vi "界面UI.vi"() -> ()   [LabVIEW 2016, in "德润DR803F超标留样.lvlib"]
uses:
  <vilib>/Utility/miscctls.llb/LVPointTypeDef.ctl
  <vilib>/Utility/config.llb/NI_LVConfig.lvlib
panel:
  out "采样瓶数":u16
  out "留样模式":T1(ring)
  out "门状态":enum16{"门关", "门开"}(ring)
  out "仪器时间":timestamp format="%<%Y/%m/%d %H:%M:%S>T"
  out "当前瓶号":u16
  out "采样器状态":enum16{"停止", "运行", "系统初始化"}(ring)
  out "采样器进程":i32(listbox)
  in  "工作进程":u16(ring) items=["清洗管路初始化", "采样瓶位置初始化", "采样瓶排空", "清洗管下降", "采样瓶清洗", "清洗管上升", "外置泵延时", "管路润洗", "进样1", "进样2", "排空管路", "采样瓶位置调整", "待机"]
  out "留样瓶满":bool
  in  "采样瓶排空":bool
  out "超标留样等待时间/s":dbl
  in  "流程停止":bool
  in  "流程启动":bool
  out "流程中":bool
  in  "外控留样设置":bool
  in  "外控留样读取":bool
  in  "设置":bool
  out "VISA resource name":refnum<visa-resource-name>="COM10" caption="VISA资源名称"
  in  "采样模式":enum16{"定时留样", "时间等比", "同步留样", "外控留样", "超标留样"}(ring)
  in  "采样启动":bool
  in  "切换运行":bool
  in  "时间校准":bool
  out "读取缓冲区":string
  out "source":string
  out "通讯":bool
  # "只在待机时启动有效"
  # "德润超标留样803F"
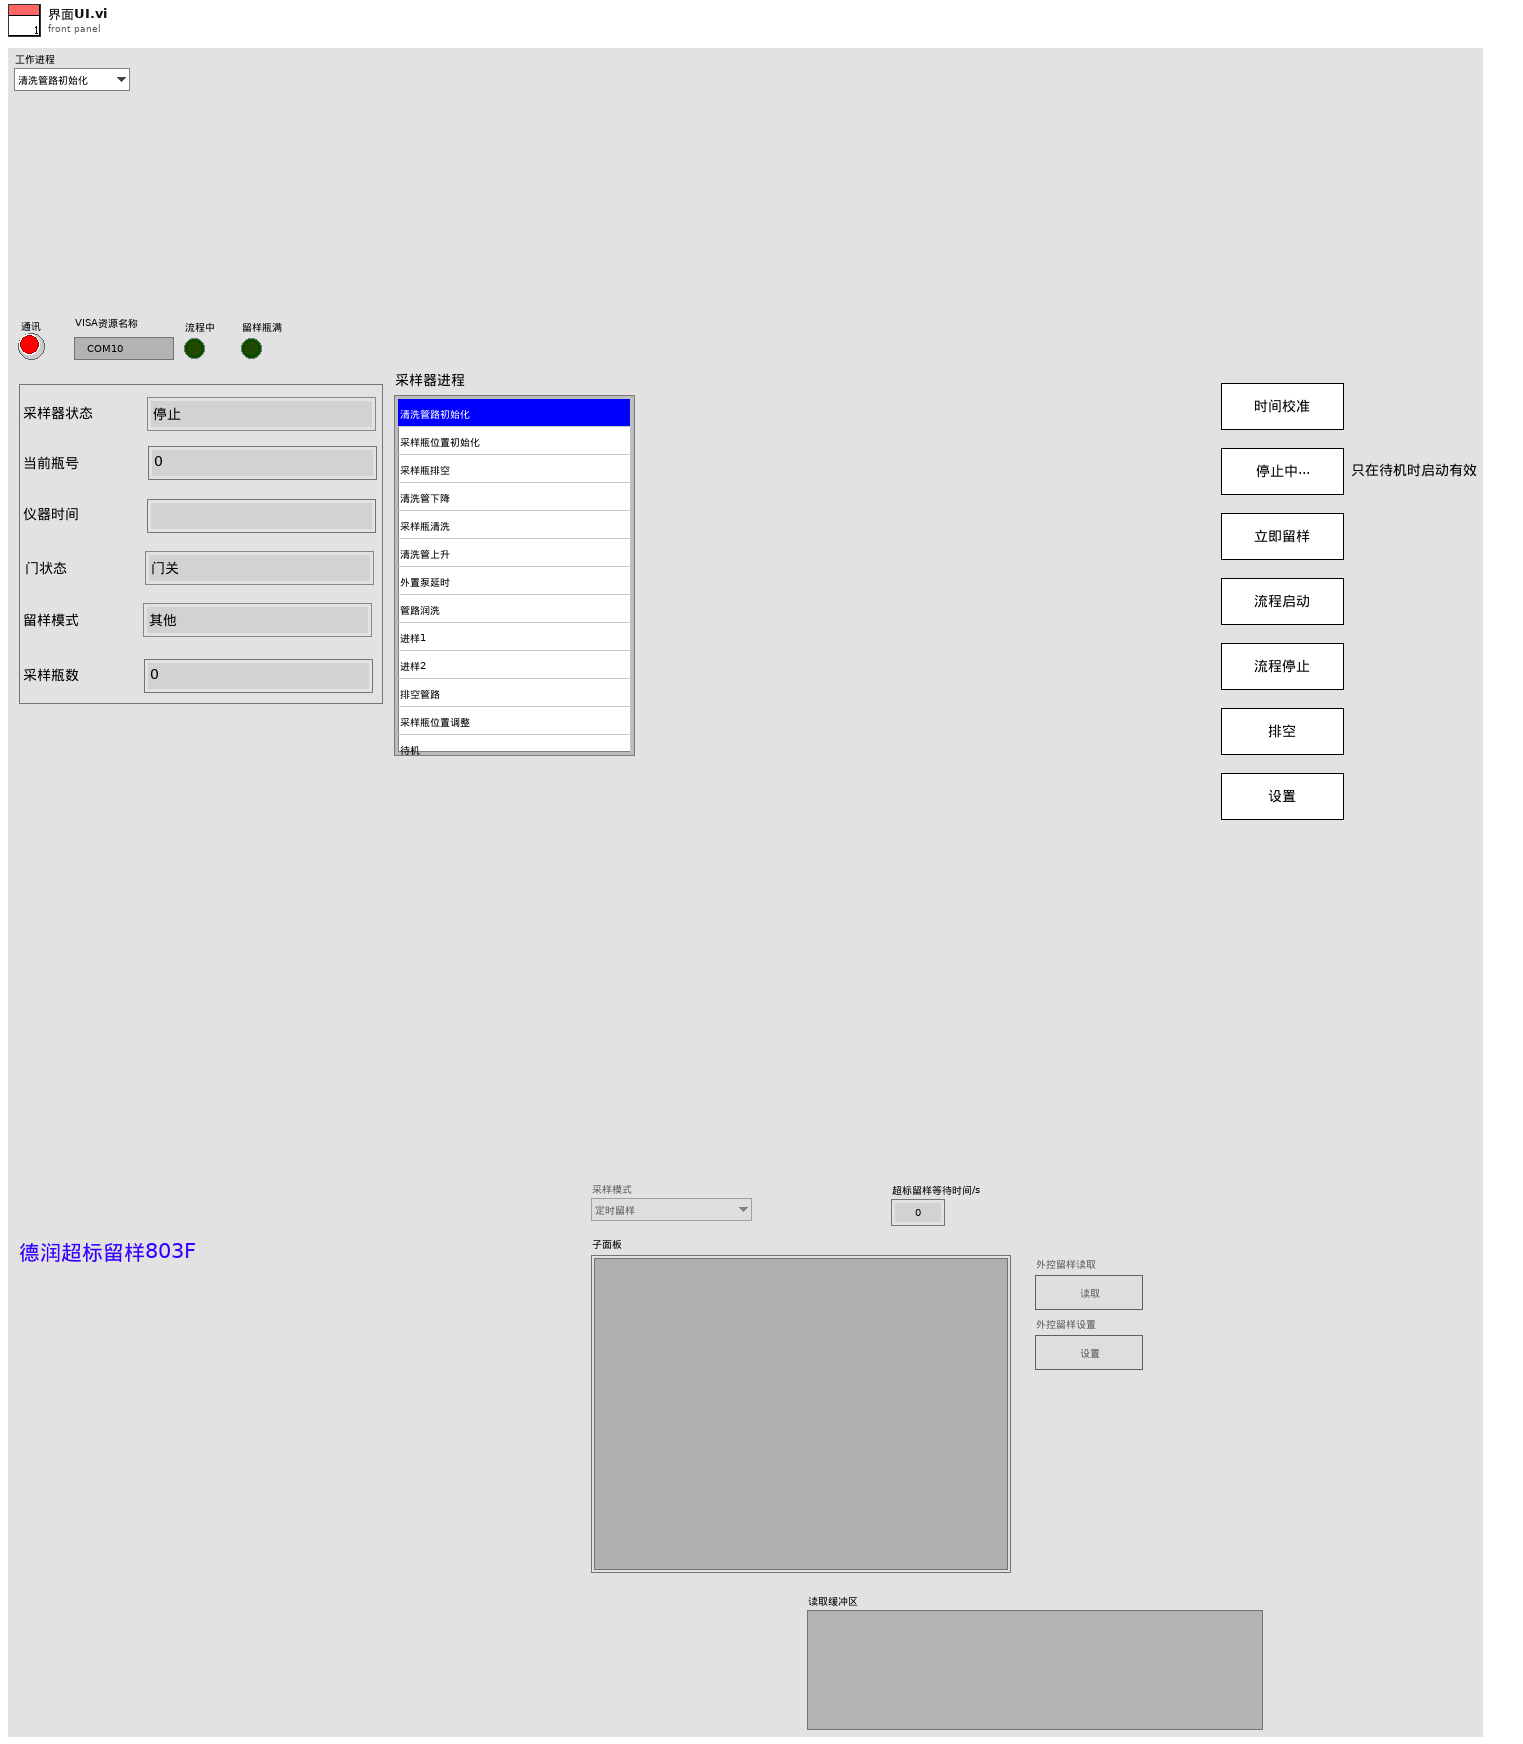
[diagram p1: front panel]
types:
  T1 = enum16{"其他", "定时留样", "时间等比例", "同步留样", "外控留样", "超标留样"}
  T2 = cluster{"枚举":enum16{"open", "read", "write", "close"}, "写入内容":string}
  T3 = cluster{"STEP":enum16{"open", "read", "write", "close"}, "写入缓冲区":string}
  T4 = typedef "LVPointTypeDef.ctl" = cluster{"Horizontal":i16, "Vertical":i16}
  T5 = typedef "NI_LVConfig.lvlib/Config Data RefNum.ctl" = refnum<k1>
  T6 = cluster{"工作状态":u16, "工作进程":u16, "仪器时间":timestamp, "采样模式":u16, "当前瓶号":dbl, "采样瓶数":dbl, "每瓶采样次数":dbl, "当前瓶已采次数":dbl, "当前瓶采样量":dbl, "采样量定量":dbl, "采样量比例":dbl, "瞬时流量":dbl, "累积流量":dbl, "外置泵状态":dbl, "采样泵状态":dbl, "采样泵方向":dbl, "采样阀":dbl, "采样瓶转盘":dbl, "排水阀":dbl, "清洗泵":dbl, "清洗管工作":dbl, "清洗管电源":dbl, "清洗管运行方向":dbl, "门状态":u16, "采水管有水检测":dbl}
  T7 = enum32{"Bad", "Idle", "Run top level", "Running"}
  T8 = cluster{"当前瓶号：":dbl, "平行样：":dbl, "留样瓶数：":dbl, "每瓶次数：":dbl, "每次留样：":dbl}
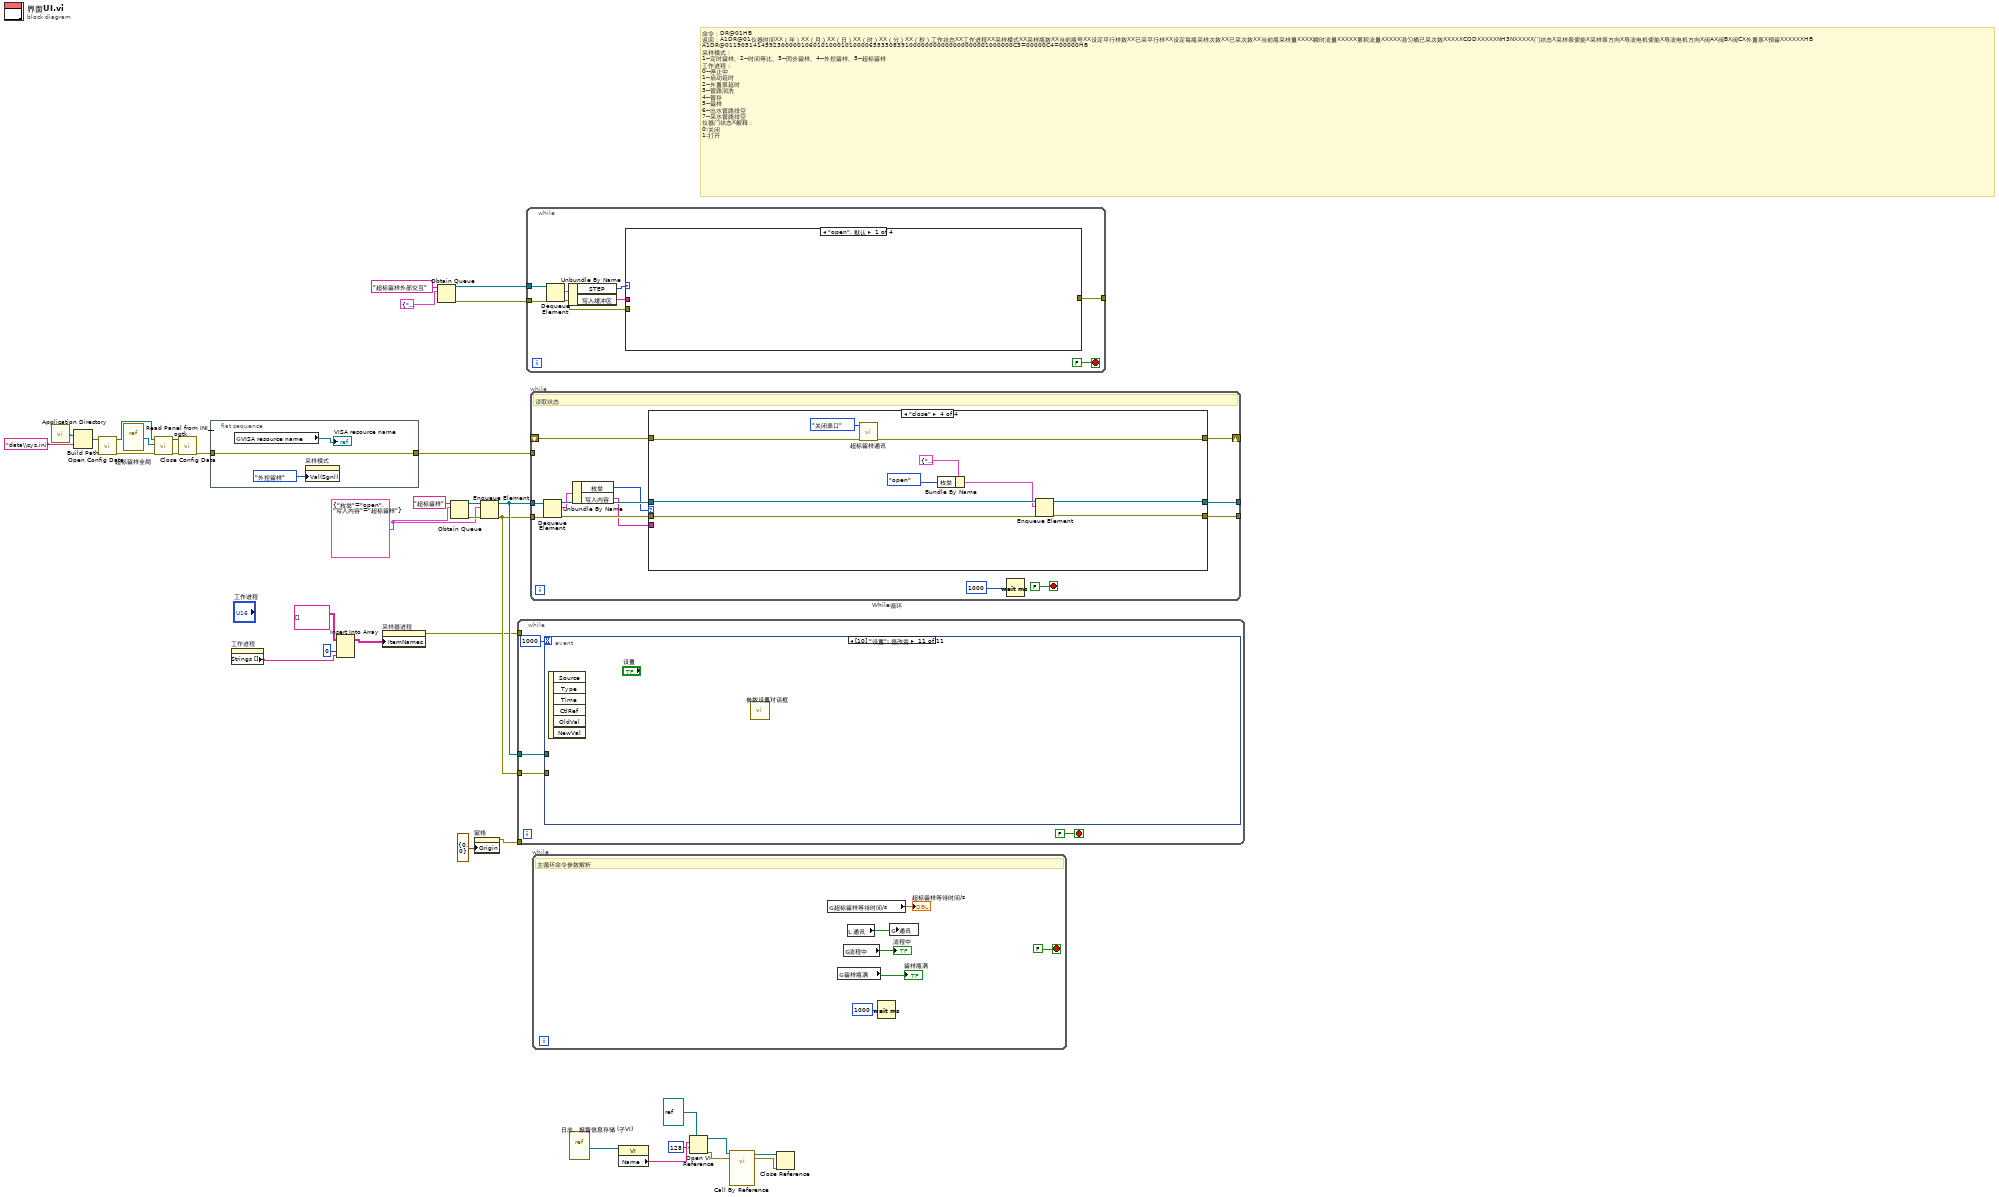
[diagram p0: block diagram]
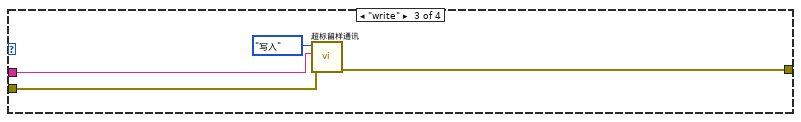
[diagram p3: hidden frame]
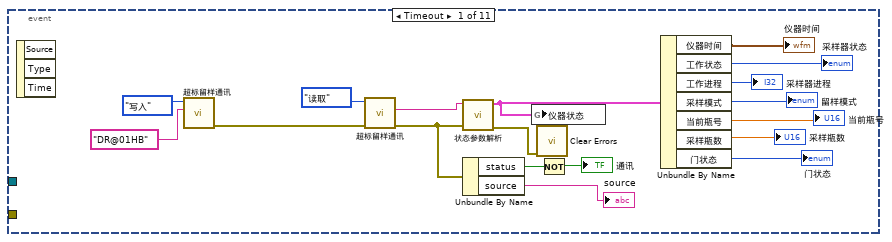
[diagram p5: hidden frame]
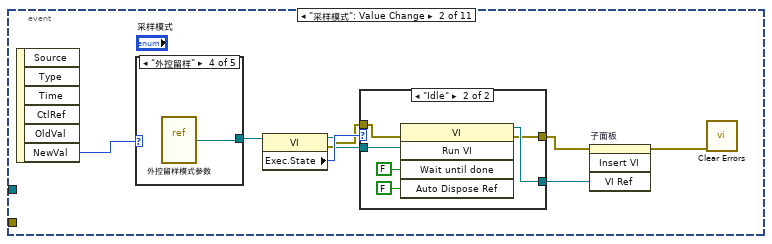
[diagram p6: hidden frame]
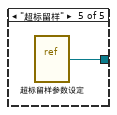
[diagram p11: hidden frame]
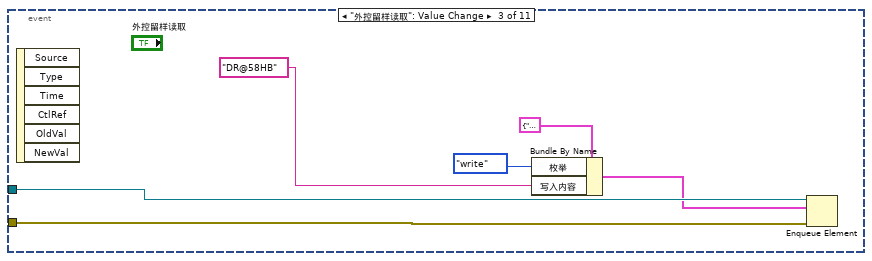
[diagram p12: hidden frame]
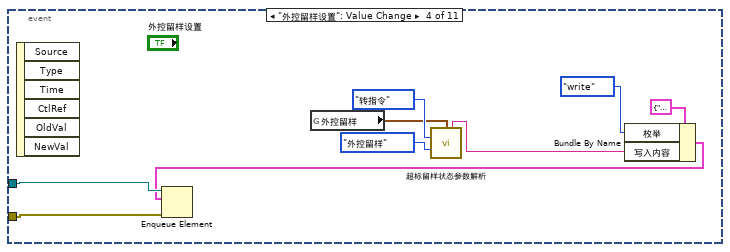
[diagram p13: hidden frame]
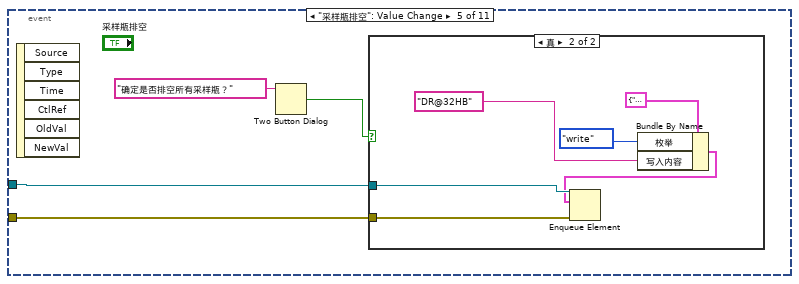
[diagram p14: hidden frame]
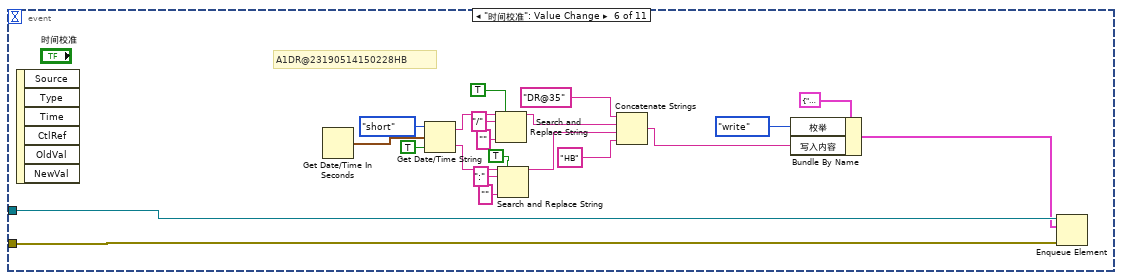
[diagram p16: hidden frame]
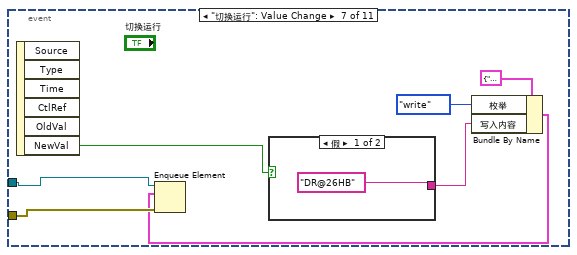
[diagram p17: hidden frame]
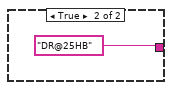
[diagram p18: hidden frame]
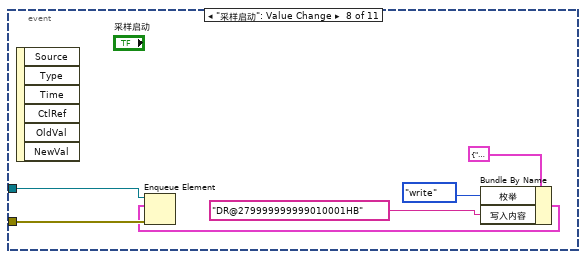
[diagram p19: hidden frame]
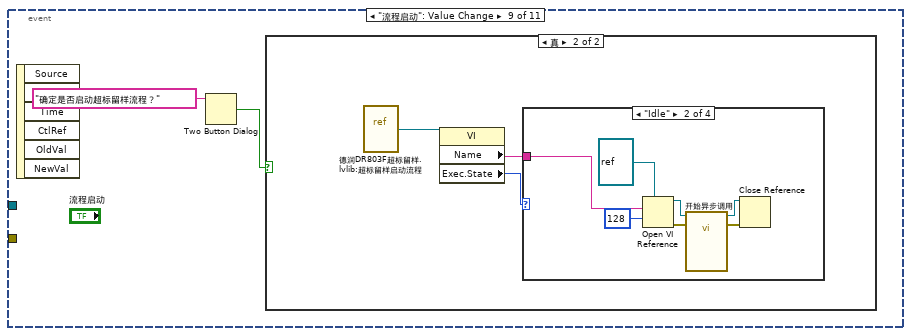
[diagram p20: hidden frame]
diagram:
  w1 = T2 {"枚举"=enum."open", "写入内容"="超标留样"}
  # "命令：DR@01HB\n返回：A1DR@01仪器时间XX（年）XX（月）XX（日）XX（时）XX（分）XX（秒）工作状态XX工作进程XX采样模式XX采样瓶数XX当前瓶号XX设定平行样数XX已采平行样XX设定每瓶采样次数XX已采次数XX当前瓶采样量XXXX瞬时流量XXXXX累积流量XXXXX混匀桶已采次数XXXXXCODXXXXXNH3NXXXXX门状态X采样泵使能X采样泵方向X导流电机使能X导流电机方向X阀AX阀BX阀CX外置泵X预留XXXXXXHB\nA1DR@011905141459230000010601010001010000655350839100000000000000000001000000C3=00000C4=00000HB\n采样模式：\n1--定时留样、2--时间等比、3--同步留样、4--外控留样、5--超标留样\n工作进程：\n0--停止中\n1--启动延时\n2--外置泵延时\n3--管路润洗\n4--管存\n5--留样\n6--出水管路排空\n7--采水管路排空\n仪器门状态X解释：\n0:关闭\n1:打开"
  n1 = call <vilib>:"Application Directory.vi"() -> ("Application Directory"=w29:path)
  n2 = Build Path(base path=w29, name or relative path="data\\sys.ini" ("名称或相对路径")) -> (appended path=w27:path)
  n3 = call <vilib>:"Open Config Data.vi"("configuration file path"=w27) -> ("error out"=w23:errorcluster, "refnum"=w26:T5)  [unwired: 8 in, 1 out]
  n4 = vi-ref "超标留样全局.vi"() -> (w25:refnum<vi>)
  n5 = call <userlib>:"Read Panel from INI__ogtk.vi"("error in (no error)"=w23, "VI ref"=w25, "refnum"=w26) -> ("error out"=w22:errorcluster, "refnum out"=w24:T5)  [unwired: 7 in]
  n6 = call <vilib>:"Close Config Data.vi"("error in (no error)"=w22, "refnum"=w24) -> ("error out"=w21:errorcluster)  [unwired: 8 in, 1 out]
  n7 = flat-sequence {
    tunnel: w21 -> [w38]
    tunnel: [w38] -> w20
    frame #0 {
      n8 = global read "超标留样全局.vi" "VISA resource name"() -> (→"VISA resource name":refnum<visa-resource-name>)
      n9 = property on="采样模式" class="Enum (严格)"("Val(Sgnl)"=enum16{"定时留样", "时间等比", "同步留样", "外控留样", "超标留样"}."外控留样" ("采样模式")) -> ()  [unwired: 2 in, 2 out]
    }
  }
  n10 = property on="工作进程" class="Ring (严格)"() -> ("Strings []"=w4:string[])  [unwired: 2 in, 2 out]
  n11 = Insert Into Array(array=string[][] [] ("字符串[]"), index (col)=0 ("禁用的索引 (列)"), new element=w4) -> (w3:string[][])  [unwired: 1 in]
  n12 = property on="采样器进程" class="MCListbox (严格)"("ItemNames"=w3) -> (error out=w2:errorcluster)  [unwired: 2 in, 1 out]
  n13 = Obtain Queue(name (unnamed)="超标留样外部交互" ("名称（未命名）"), element data type=T3 {"STEP"=enum."write", "写入缓冲区"="ª\u0006\u0000\u0000P`\u00000»"}) -> (queue out=w18:refnum<queue>, error out=w17:errorcluster)  [unwired: 3 in, 1 out]
  n14 = Obtain Queue(name (unnamed)="超标留样" ("名称（未命名）"), element data type=w1) -> (queue out=w34:refnum<queue>, error out=w33:errorcluster)  [unwired: 3 in, 1 out]
  n15 = property on="窗格" class="Pane"("Origin"=T4 {"Horizontal"=0, "Vertical"=0} ("原点")) -> (error out=w7:errorcluster)  [unwired: 2 in, 1 out]
  n16 = Enqueue Element(queue=w34, element=w1, error in (no error)=w33) -> (queue out=w32:refnum<queue>, error out=w31:errorcluster)  [unwired: 1 in, 1 out]
  n17 = while {
    tunnel: w32 -> [w41]
    tunnel: w31 -> [w40]
    tunnel: w7 -> [_]
    tunnel: w2 -> [_]
    stop <- FALSE stop-if-true
    n18 = event shown="[10] \"设置\": 值改变" {
      selector: _ -> [_ _ _ _ _ _ _ _ _ _ _]
      dyn-events: _ -> [_ _ _ _ _ _ _ _ _ _ _]
      timeout: 1000 -> [_ _ _ _ _ _ _ _ _ _ _]
      tunnel: w41 -> [_ _ w83 w93 w97 w124 w131 w139 _ w153 _]
      tunnel: w40 -> [_ _ w84 w92 w96 w123 w130 w138 _ w152 _]
      event Timeout {
        n19 = event-data() -> ()  [unwired: 1 in, 3 out]
        n20 = call "超标留样通讯.vi"("写入缓冲区"="DR@01HB", "功能输入"=enum16{"打开串口", "写入", "读取", "关闭串口"}."写入") -> ("error out"=w60:errorcluster)  [unwired: 7 in, 2 out]
        n21 = call "超标留样通讯.vi"("error in (no error)"=w60, "功能输入"=enum16{"打开串口", "写入", "读取", "关闭串口"}."读取") -> ("error out"=w59:errorcluster, "读取缓冲区"=w58:string)  [unwired: 7 in, 1 out]
        n22 = call "状态参数解析.vi"("error in (no error)"=w59, "字符串"=w58) -> ("error out"=w43:errorcluster, "簇"=w51:T6)  [unwired: 8 in]
        n23 = Unbundle By Name(w59) -> ("status"=w52:bool, "source"=→"source":string)
        n24 = global write "超标留样全局.vi" "仪器状态"(w51) -> ()
        n25 = call <vilib>:"Clear Errors.vi"("error in (no error)"=w43) -> ()  [unwired: 5 in, 2 out]
        n26 = Not(x=w52) -> (.not. x?=→"通讯":bool)
        n27 = Unbundle By Name(w51) -> ("仪器时间"=→"仪器时间":timestamp, "工作状态"=→"采样器状态":u16, "工作进程"=→"采样器进程":u16, "采样模式"=→"留样模式":u16, "当前瓶号"=→"当前瓶号":dbl, "采样瓶数"=→"采样瓶数":dbl, "门状态"=→"门状态":u16)
      }
      event "采样模式": Value Change {
        n28 = event-data() -> ("NewVal"=w68:enum16{"定时留样", "时间等比", "同步留样", "外控留样", "超标留样"})  [unwired: 1 in, 5 out]
        n29 = case shown="\"外控留样\"" w68 {
          tunnel: [_ _ _ w77 w78] -> w67
          frame "定时留样", Default {
          }
          frame "时间等比" {
          }
          frame "同步留样" {
          }
          frame "外控留样" {
            n30 = vi-ref "外控留样模式参数.vi"() -> (w77:refnum<vi>)
          }
          frame "超标留样" {
            n31 = vi-ref "超标留样参数设定.vi"() -> (w78:refnum<vi>)
          }
        }
        n32 = property class="VI"(reference=w67) -> (reference out=w65:refnum<vi>, error out=w63:errorcluster, "Exec.State"=w66:T7)  [unwired: 1 in]
        n33 = case shown="\"Idle\"" w66 {
          tunnel: w65 -> [w70 w76]
          tunnel: [w70 w73] -> w64
          tunnel: w63 -> [w69 w72]
          tunnel: [w69 w71] -> w62
          frame "Bad", Default {
          }
          frame "Idle" {
            n34 = invoke class="VI" method="Run VI"(reference=w76, error in=w72, "Wait until done"=FALSE ("结束前等待"), "Auto Dispose Ref"=FALSE ("自动销毁引用")) -> (reference out=w73:refnum<vi>, error out=w71:errorcluster)  [unwired: 1 in, 3 out]
          }
        }
        n35 = invoke on="子面板" class="SubPnl" method="Insert VI"(error in=w62, "VI Ref"=w64) -> (error out=w61:errorcluster)  [unwired: 2 in, 3 out]
        n36 = call <vilib>:"Clear Errors.vi"("error in (no error)"=w61) -> ()  [unwired: 5 in, 2 out]
      }
      event "外控留样读取": Value Change {
        n37 = event-data() -> ()  [unwired: 1 in, 6 out]
        n38 = Bundle By Name(cluster=T2 {"枚举"=enum."open", "写入内容"="超标留样"}, "枚举"=enum16{"open", "read", "write", "close"}."write" ("元素"), "写入内容"="DR@58HB") -> (w79:T2)
        n39 = Enqueue Element(queue=w83, element=w79, error in (no error)=w84) -> ()  [unwired: 1 in, 3 out]
      }
      event "外控留样设置": Value Change {
        n40 = event-data() -> ()  [unwired: 1 in, 6 out]
        n41 = global read "超标留样全局.vi" "外控留样"() -> (w89:T8)
        n42 = call "超标留样状态参数解析.vi"("外控留样"=w89, "解析/转指令"=enum16{"解析", "转指令"}."转指令", "模式选择"=enum16{"外控留样", "超标留样"}."外控留样") -> ("输出字符串"=w86:string)  [unwired: 11 in, 1 out]
        n43 = Bundle By Name(cluster=T2 {"枚举"=enum."open", "写入内容"="超标留样"}, "枚举"=enum16{"open", "read", "write", "close"}."write" ("元素"), "写入内容"=w86) -> (w85:T2)
        n44 = Enqueue Element(queue=w93, element=w85, error in (no error)=w92) -> ()  [unwired: 1 in, 3 out]
      }
      event "采样瓶排空": Value Change {
        n45 = event-data() -> ()  [unwired: 1 in, 6 out]
        n46 = Two Button Dialog(message="确定是否排空所有采样瓶？" ("消息")) -> (T button?=w94:bool)  [unwired: 2 in]
        n47 = case shown="真" w94 {
          tunnel: w97 -> [_ w103]
          tunnel: w96 -> [_ w102]
          frame False {
          }
          frame True {
            n48 = Bundle By Name(cluster=T2 {"枚举"=enum."open", "写入内容"="超标留样"}, "枚举"=enum16{"open", "read", "write", "close"}."write" ("元素"), "写入内容"="DR@32HB") -> (w98:T2)
            n49 = Enqueue Element(queue=w103, element=w98, error in (no error)=w102) -> ()  [unwired: 1 in, 3 out]
          }
        }
      }
      event "时间校准": Value Change {
        # "A1DR@23190514150228HB"
        n50 = event-data() -> ()  [unwired: 1 in, 6 out]
        n51 = Get Date/Time In Seconds() -> (seconds since 1Jan1904=w119:timestamp)
        n52 = Get Date/Time String(date format (0)=enum16{"short", "long", "abbreviated"}."short" ("日期格式(0)"), seconds (now)=w119, want seconds? (F)=TRUE ("需要秒？(F)")) -> (date string=w118:string, time string=w111:string)
        n53 = Search and Replace String(replace all?=TRUE ("替换全部？(F)"), input string=w118, search string="/" ("搜索字符串"), replace string="" ("替换字符串(\"\")")) -> (result string=w110:string)  [unwired: 4 in, 3 out]
        n54 = Search and Replace String(replace all?=TRUE ("替换全部？(F)"), input string=w111, search string=":" ("搜索字符串"), replace string="" ("替换字符串(\"\")")) -> (result string=w109:string)  [unwired: 4 in, 3 out]
        n55 = Concatenate Strings("DR@35" ("写入缓冲区"), w110, w109, "HB" ("写入缓冲区")) -> (w105:string)
        n56 = Bundle By Name(cluster=T2 {"枚举"=enum."open", "写入内容"="超标留样"}, "枚举"=enum16{"open", "read", "write", "close"}."write" ("元素"), "写入内容"=w105) -> (w104:T2)
        n57 = Enqueue Element(queue=w124, element=w104, error in (no error)=w123) -> ()  [unwired: 1 in, 3 out]
      }
      event "切换运行": Value Change {
        n58 = event-data() -> ("NewVal"=w127:bool)  [unwired: 1 in, 5 out]
        n59 = case shown="假" w127 {
          tunnel: ["DR@26HB" ("写入缓冲区") "DR@25HB"] -> w126
          frame False {
          }
          frame True {
          }
        }
        n60 = Bundle By Name(cluster=T2 {"枚举"=enum."open", "写入内容"="超标留样"}, "枚举"=enum16{"open", "read", "write", "close"}."write" ("元素"), "写入内容"=w126) -> (w125:T2)
        n61 = Enqueue Element(queue=w131, element=w125, error in (no error)=w130) -> ()  [unwired: 1 in, 3 out]
      }
      event "采样启动": Value Change {
        n62 = event-data() -> ()  [unwired: 1 in, 6 out]
        n63 = Bundle By Name(cluster=T2 {"枚举"=enum."open", "写入内容"="超标留样"}, "枚举"=enum16{"open", "read", "write", "close"}."write" ("元素"), "写入内容"="DR@279999999999010001HB") -> (w134:T2)
        n64 = Enqueue Element(queue=w139, element=w134, error in (no error)=w138) -> ()  [unwired: 1 in, 3 out]
      }
      event "流程启动": Value Change {
        n65 = event-data() -> ()  [unwired: 1 in, 6 out]
        n66 = Two Button Dialog(message="确定是否启动超标留样流程？" ("消息")) -> (T button?=w140:bool)  [unwired: 2 in]
        n67 = case shown="真" w140 {
          frame False {
          }
          frame True {
            n68 = vi-ref "德润DR803F超标留样.lvlib:超标留样启动流程.vi"() -> (w142:refnum<vi>)
            n69 = property class="VI"(reference=w142) -> ("Name"=w143:string, "Exec.State"=w144:T7)  [unwired: 1 in, 2 out]
            n70 = case shown="\"Idle\"" w144 {
              tunnel: w143 -> [_ w147 _ _]
              frame "Bad", Default {
              }
              frame "Idle" {
                n71 = Open VI Reference(type specifier VI Refnum (for type only)=refnum<vi> refnum ("类型说明符VI引用句柄（仅用于类型）"), vi path=w147, options=128 ("选项")) -> (vi reference=w151:refnum<vi>, error out=w146:errorcluster)  [unwired: 3 in]
                n72 = call-by-ref "开始异步调用"(reference=w151, error in=w146) -> (reference out=w150:refnum<vi>, error out=w145:errorcluster)  [unwired: 12 in]
                n73 = Close Reference(reference=w150, error in (no error)=w145) -> ()  [unwired: 1 out]
              }
              frame "Run top level" {
              }
              frame "Running" {
              }
            }
          }
        }
      }
      event "流程停止": Value Change {
        n74 = event-data() -> ()  [unwired: 1 in, 6 out]
        n75 = Two Button Dialog(message="确定是否停止超标留样流程并排空当前瓶？" ("消息")) -> (T button?=w154:bool)  [unwired: 2 in]
        n76 = case shown="真" w154 {
          tunnel: w153 -> [_ w161]
          tunnel: w152 -> [_ w160]
          frame False {
          }
          frame True {
            n77 = Obtain Notifier(name (unnamed)="超标留样流程" ("名称（未命名）"), notification data type=FALSE ("采样完成")) -> (notifier out=w166:refnum<notifier>, error out=w165:errorcluster)  [unwired: 2 in, 1 out]
            n78 = Send Notification(notification=TRUE ("通知"), notifier=w166, error in (no error)=w165) -> (notifier out=w163:refnum<notifier>, error out=w162:errorcluster)
            n79 = Release Notifier(notifier=w163, error in (no error)=w162) -> ()  [unwired: 1 in, 3 out]
            n80 = Bundle By Name(cluster=T2 {"枚举"=enum."open", "写入内容"="超标留样"}, "枚举"=enum16{"open", "read", "write", "close"}."write" ("元素"), "写入内容"="DR@26HB" ("写入缓冲区")) -> (w156:T2)
            n81 = Enqueue Element(queue=w161, element=w156, error in (no error)=w160) -> ()  [unwired: 1 in, 3 out]
          }
        }
      }
      event "设置": Value Change {
        n82 = event-data() -> ()  [unwired: 1 in, 6 out]
        n83 = call "参数设置对话框.vi"() -> ()  [unwired: 12 in]
      }
    }
  }
  n84 = while {
    tunnel: w18 -> [w176]
    tunnel: w17 -> [w175]
    tunnel: [w169] -> _
    stop <- FALSE stop-if-true
    n85 = Dequeue Element(queue=w176, error in (no error)=w175) -> (element=w173:T3, error out=w170:errorcluster)  [unwired: 1 in, 2 out]
    n86 = Unbundle By Name(w173) -> ("STEP"=w172:enum16{"open", "read", "write", "close"}, "写入缓冲区"=w171:string)
    n87 = case shown="\"open\", 默认" w172 {
      tunnel: w171 -> [_ _ w180 _]
      tunnel: w170 -> [_ _ w178 _]
      tunnel: [_ _ w177 _] -> w169
      frame "open", Default {
      }
      frame "read" {
      }
      frame "write" {
        n88 = call "超标留样通讯.vi"("error in (no error)"=w178, "写入缓冲区"=w180, "功能输入"=enum16{"打开串口", "写入", "读取", "关闭串口"}."写入") -> ("error out"=w177:errorcluster)  [unwired: 6 in, 2 out]
      }
      frame "close" {
      }
    }
  }
  n89 = while "While循环" {
    tunnel: w32 -> [w191]
    tunnel: w31 -> [w190]
    tunnel: [w187] -> _
    tunnel: [w186] -> _
    shift-right: [w184] -> _
    shift-left: _ -> [w185]
    tunnel: w20 -> [_]
    stop <- FALSE stop-if-true
    # "读取状态"
    n90 = Dequeue Element(queue=w191, error in (no error)=w190) -> (queue out=w189:refnum<queue>, element=w183:T2, error out=w188:errorcluster)  [unwired: 1 in, 1 out]
    n91 = Unbundle By Name(w183) -> ("枚举"=w182:enum16{"open", "read", "write", "close"}, "写入内容"=w181:string)
    n92 = case shown="\"close\"" w182 {
      tunnel: [w197 w200 w225 w238] -> w184
      tunnel: w189 -> [w196 w203 w230 w237]
      tunnel: w188 -> [w195 w202 w229 w236]
      tunnel: [w196 w203 w228 w235] -> w187
      tunnel: [w195 w202 w227 w234] -> w186
      tunnel: w185 -> [_ w205 w226 w240]
      tunnel: w181 -> [_ w199 w221 _]
      frame "open", Default {
        (unwired) refnum<visa-resource-name> "COM2" ("VISA resource name")
        n93 = global read "超标留样全局.vi" "VISA resource name"() -> (w194:refnum<visa-resource-name>)
        n94 = call "超标留样通讯.vi"("VISA resource name"=w194, "功能输入"=enum16{"打开串口", "写入", "读取", "关闭串口"}."打开串口") -> ("error out"=w197:errorcluster)  [unwired: 7 in, 2 out]
      }
      frame "read" {
        n95 = call "超标留样通讯.vi"("error in (no error)"=w205, "功能输入"=enum16{"打开串口", "写入", "读取", "关闭串口"}."读取") -> ("error out"=w200:errorcluster, "读取缓冲区"=w201:string)  [unwired: 7 in, 1 out]
        "读取缓冲区" <- w201
        n96 = case shown="\"DR@58HB\"" w199 {
          tunnel: w201 -> [w206 w213 _]
          frame "超标留样读取" {
            n97 = flat-sequence {
              tunnel: w206 -> [w209]
              frame #0 {
                n98 = call "超标留样状态参数解析.vi"("输入字符串"=w209, "解析/转指令"=enum16{"解析", "转指令"}."解析", "模式选择"=enum16{"外控留样", "超标留样"}."超标留样") -> ()  [unwired: 11 in, 2 out]
              }
              frame #1 {
                n99 = global write "超标留样全局.vi" "读取更新"(TRUE ("读取更新")) -> ()
              }
              frame #2 {
                n100 = Wait (ms)(milliseconds to wait=u32 500 ("等待时间（毫秒）")) -> ()  [unwired: 1 out]
              }
              frame #3 {
                n101 = global write "超标留样全局.vi" "读取更新"(FALSE ("读取更新")) -> ()
              }
            }
          }
          frame "DR@58HB" {
            n102 = flat-sequence {
              tunnel: w213 -> [w214]
              frame #0 {
                n103 = call "超标留样状态参数解析.vi"("输入字符串"=w214, "解析/转指令"=enum16{"解析", "转指令"}."解析", "模式选择"=enum16{"外控留样", "超标留样"}."外控留样") -> ()  [unwired: 11 in, 2 out]
              }
              frame #1 {
                n104 = global write "超标留样全局.vi" "外控留样读取更新"(TRUE ("读取更新")) -> ()
              }
              frame #2 {
                n105 = Wait (ms)(milliseconds to wait=u32 500 ("等待时间（毫秒）")) -> ()  [unwired: 1 out]
              }
              frame #3 {
                n106 = global write "超标留样全局.vi" "外控留样读取更新"(FALSE ("读取更新")) -> ()
              }
            }
          }
          frame "超标留样设置", Default {
          }
        }
      }
      frame "write" {
        n107 = call "超标留样通讯.vi"("error in (no error)"=w226, "写入缓冲区"=w221, "功能输入"=enum16{"打开串口", "写入", "读取", "关闭串口"}."写入") -> ("error out"=w225:errorcluster)  [unwired: 6 in, 2 out]
        n108 = Bundle By Name(cluster=T2 {"枚举"=enum."open", "写入内容"="超标留样"}, "枚举"=enum16{"open", "read", "write", "close"}."read" ("元素"), "写入内容"=w221) -> (w220:T2)
        n109 = Enqueue Element(queue=w230, element=w220, error in (no error)=w229) -> (queue out=w228:refnum<queue>, error out=w227:errorcluster)  [unwired: 1 in, 1 out]
      }
      frame "close" {
        n110 = call "超标留样通讯.vi"("error in (no error)"=w240, "功能输入"=enum16{"打开串口", "写入", "读取", "关闭串口"}."关闭串口") -> ("error out"=w238:errorcluster)  [unwired: 7 in, 2 out]
        n111 = Bundle By Name(cluster=T2 {"枚举"=enum."open", "写入内容"="超标留样"}, "枚举"=enum16{"open", "read", "write", "close"}."open" ("元素")) -> (w231:T2)
        n112 = Enqueue Element(queue=w237, element=w231, error in (no error)=w236) -> (queue out=w235:refnum<queue>, error out=w234:errorcluster)  [unwired: 1 in, 1 out]
      }
    }
    n113 = Wait (ms)(milliseconds to wait=u32 1000 ("等待时间（毫秒）")) -> ()  [unwired: 1 out]
  }
  n114 = while {
    stop <- FALSE stop-if-true
    # "主循环命令参数解析"
    n115 = global read "超标留样全局.vi" "超标留样等待时间/s"() -> (→"超标留样等待时间/s":dbl)
    n116 = global read "超标留样全局.vi" "留样瓶满"() -> (→"留样瓶满":bool)
    n117 = global read "超标留样全局.vi" "流程中"() -> (→"流程中":bool)
    n118 = local read "通讯"() -> (w244:bool)
    n119 = Wait (ms)(milliseconds to wait=u32 1000 ("等待时间（毫秒）")) -> ()  [unwired: 1 out]
    n120 = global write "超标留样全局.vi" "通讯"(w244) -> ()
  }
  n121 = vi-ref "日志、报警信息存储 (子VI).vi"() -> (w15:refnum<vi>)
  n122 = property class="VI"(reference=w15) -> ("Name"=w14:string)  [unwired: 1 in, 2 out]
  n123 = Open VI Reference(type specifier VI Refnum (for type only)=refnum<vi> refnum ("类型说明符VI引用句柄（仅用于类型）"), vi path=w14, options=128 ("选项")) -> (vi reference=w12:refnum<vi>, error out=w10:errorcluster)  [unwired: 3 in]
  n124 = call-by-ref "?"(reference=w12, error in=w10) -> (reference out=w9:refnum<vi>, error out=w8:errorcluster)  [unwired: 12 in]
  n125 = Close Reference(reference=w9, error in (no error)=w8) -> ()  [unwired: 1 out]
